vi "Setting.vi"() -> ()   [LabVIEW 2015]
uses:
  Control/Setting_Control_Main Action.ctl
  <vilib>/vision/Measure.llb/Edge Polarity.ctl
  <vilib>/Utility/miscctls.llb/LVPointTypeDef.ctl
  <vilib>/userdefined/High Color/IMAQdx.ctl
panel:
  out "狀態：":string
  out "群組：":string
  out "帳號：":string
  in  "物料名稱":enum16{"Tressel", "Diablo"}(ring)
  in  "匯入圖片":bool
  in  "邊參數L":T1={"Search Direction"=0, "Edge Polarity"=0, "Kernel Size"=3, "Width"=3, "Minimum Edge Strength"=10.0} {"Minimum Edge Strength" format="%.2f"; "Width" step=2; "Kernel Size" step=2; "Edge Polarity" items=["All Edges", "Rising Edges", "Falling Edges"]; "Search Direction" items=["Left to Right", "Right to Left", "Top to Bottom", "Bottom to Top"]}
  in  "邊參數R":T1={"Search Direction"=0, "Edge Polarity"=0, "Kernel Size"=3, "Width"=3, "Minimum Edge Strength"=10.0} {"Minimum Edge Strength" format="%.2f"; "Width" step=2; "Kernel Size" step=2; "Edge Polarity" items=["All Edges", "Rising Edges", "Falling Edges"]; "Search Direction" items=["Left to Right", "Right to Left", "Top to Bottom", "Bottom to Top"]}
  in  "樣本比對參數R":T3={"方法"=1, "分數"=800.0, "起始角度"=-5.0, "結束角度"=5.0} {"結束角度" min=-180 max=180 step=5; "方法" items=["快速比對"=1, "精準比對"=2]; "起始角度" min=-180 max=180 step=5}
  in  "樣本比對參數L":T3={"方法"=1, "分數"=800.0, "起始角度"=-5.0, "結束角度"=5.0} {"結束角度" min=-180 max=180 step=5; "方法" items=["快速比對"=1, "精準比對"=2]; "起始角度" min=-180 max=180 step=5}
  in  "確認檢測項目":bool
  in  "檢測項目":T4
  out "Patttern_R":T5(plugin-control)
  out "Patttern_L":T5(plugin-control)
  out "Image":T5(plugin-control)
  in  "離開":bool
  in  "連續測試":bool
  in  "單步測試":bool
  in  "連續取像":bool
  in  "取像":bool
  out "Set action":T6
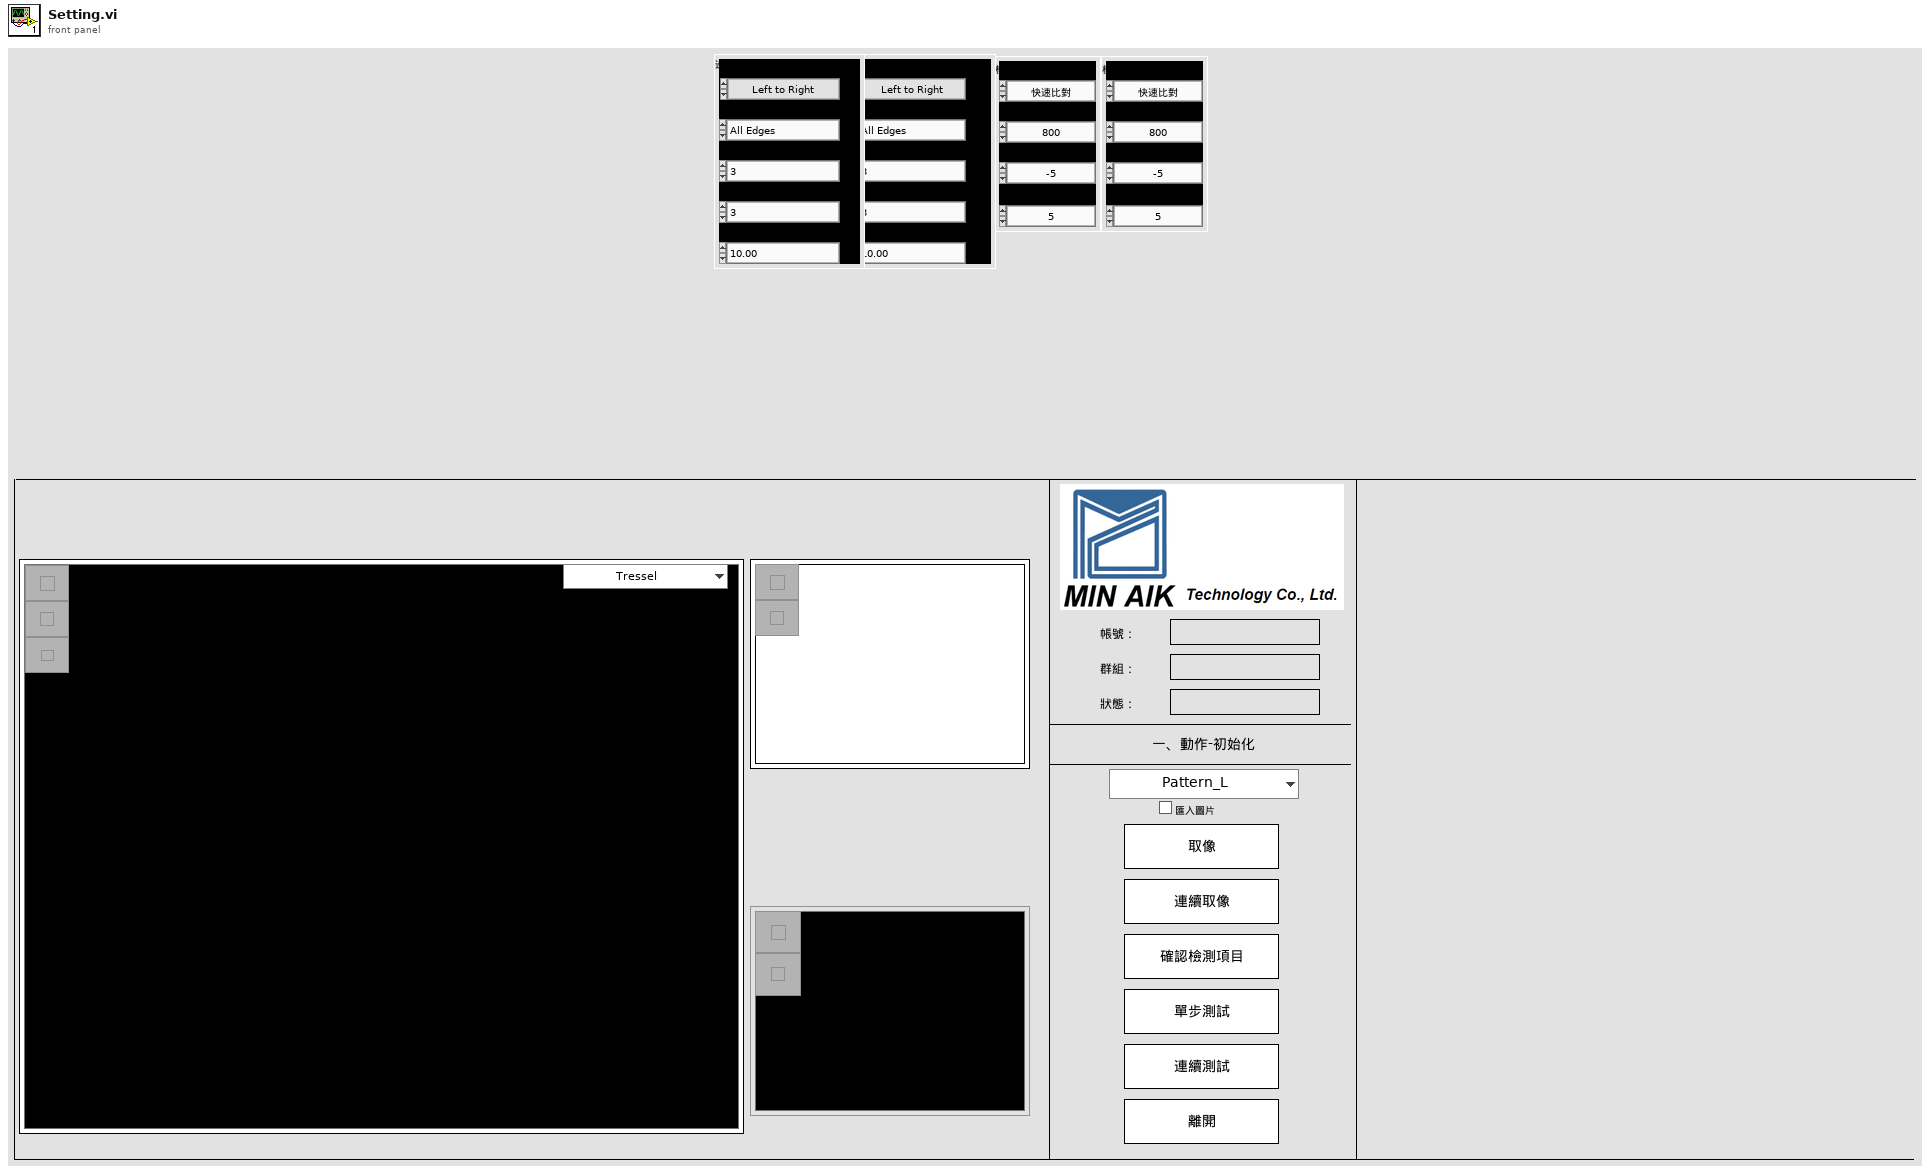
[diagram p1: front panel]
types:
  T1 = typedef "Setting_Control_Line Paremeter.ctl" = cluster{"Search Direction":u32, "Edge Polarity":T2, "Kernel Size":u32, "Width":u32, "Minimum Edge Strength":sgl}
  T2 = typedef "Edge Polarity.ctl" = u32
  T3 = typedef "Setting_Control_Pattern Paremeter.ctl" = cluster{"方法":u16, "分數":sgl, "起始角度":sgl, "結束角度":sgl}
  T4 = typedef "Setting_Control_檢測項目.ctl" = enum16{"Pattern_L", "Match_L", "Pattern_R", "Match_R", "找邊_L", "找邊R"}
  T5 = typedef "IMAQ Image.ctl" = refnum<image>
  T6 = typedef "Setting_Control_Main Action.ctl" = enum16{"一、動作-初始化", "二、動作-單次取像", "三、動作-連續取像", "四、動作-單步測試", "五、動作-連續測試", "六、動作-離開", "1.0 功能-IO控制", "       1.1 IO-初始化", "       1.2 Set Point(EOT On)", "       1.3Set Point(EOT Off)", "       1.4Get Point(SOT)", "2.0功能-相機控制", "       2.1相機-初始化", "       2.2相機-取像", "       2.3相機-關閉", "3.0功能-影像控制", "       3.1影像-初始化", "       3.2影像-更新影像", "       3.3影像-儲存影像", "4.0功能-檢測", "       4.1檢測-初始化", "      4.2浪代-浪代", "             4.2.1浪代-Pattern_L", "             4.2.2浪代-Match_L", "             4.2.3浪代-Pattern_R", "             4.2.4浪代-Match_R", "             4.2.5檢測-找邊_L", "             4.2.6檢測-找邊_R", "5.0功能-雷射控制", "      5.1雷射-初始化", "      5.2雷射-寫入數值", "      5.3雷射-讀出數值", "      5.4雷射-雷射觸發", "      5.5雷射-關閉", "6.0功能-檔案", "       6.1檔案-初始化", "       6.2檔案-儲存檔案", "       6.3檔案-開啟檔案", "7.0 錯誤", "8.0等待", "       8.1等待(計算時間)", "9.0離開", "10.0功能-機台驗證", "      10.1機台驗證-初始化", "      10.2機台驗證-檢測", "11.0對話視窗"}
  T7 = typedef "LVPointTypeDef.ctl" = cluster{"Horizontal":i16, "Vertical":i16}
  T8 = typedef "IMAQdx.ctl" = refnum<k21>
  T9 = typedef "action_camera.ctl" = enum16{"初始化", "取像", "匯入影像", "結束"}
  T10 = typedef "Image action.ctl" = enum16{"初始化", "創造記憶體", "寫入圖片", "讀取圖片", "刪除圖片", "等待"}
  T11 = cluster{"邊參數R":T1, "ROI":cluster{"Global Rectangle":i32[], "Contours":cluster{"Contour Type":u32, "ROI Type":u32, "Points":i32[]}[]}}
  T12 = cluster{"邊參數L":T1, "ROI":cluster{"Global Rectangle":i32[], "Contours":cluster{"Contour Type":u32, "ROI Type":u32, "Points":i32[]}[]}}
  T13 = typedef "IMAQ Coordinate System" = cluster{"Reference System":cluster{"Origin":cluster{"X":sgl, "Y":sgl}, "Angle (deg)":sgl, "Axis Reference":u32}, "Measurement System":cluster{"Origin":cluster{"X":sgl, "Y":sgl}, "Angle (deg)":sgl, "Axis Reference":u32}}
  T14 = cluster{"ROI":cluster{"Global Rectangle":i32[], "Contours":cluster{"Contour Type":u32, "ROI Type":u32, "Points":i32[]}[]}, "樣本比對參數R":T3, "Coordinate System Out":T13}
  T15 = cluster{"樣本比對參數L":T3, "ROI":cluster{"Global Rectangle":i32[], "Contours":cluster{"Contour Type":u32, "ROI Type":u32, "Points":i32[]}[]}, "Coordinate System Out":T13}
  T16 = typedef "Action_Data.ctl" = enum16{"Initialize", "Get Data", "Set Data", "Delete Data", "Idle"}
  T17 = typedef "Image Type" = u32
  T18 = cluster{"Global Rectangle":i32[], "Contours":cluster{"Contour Type":u32, "ROI Type":u32, "Points":i32[]}[]}
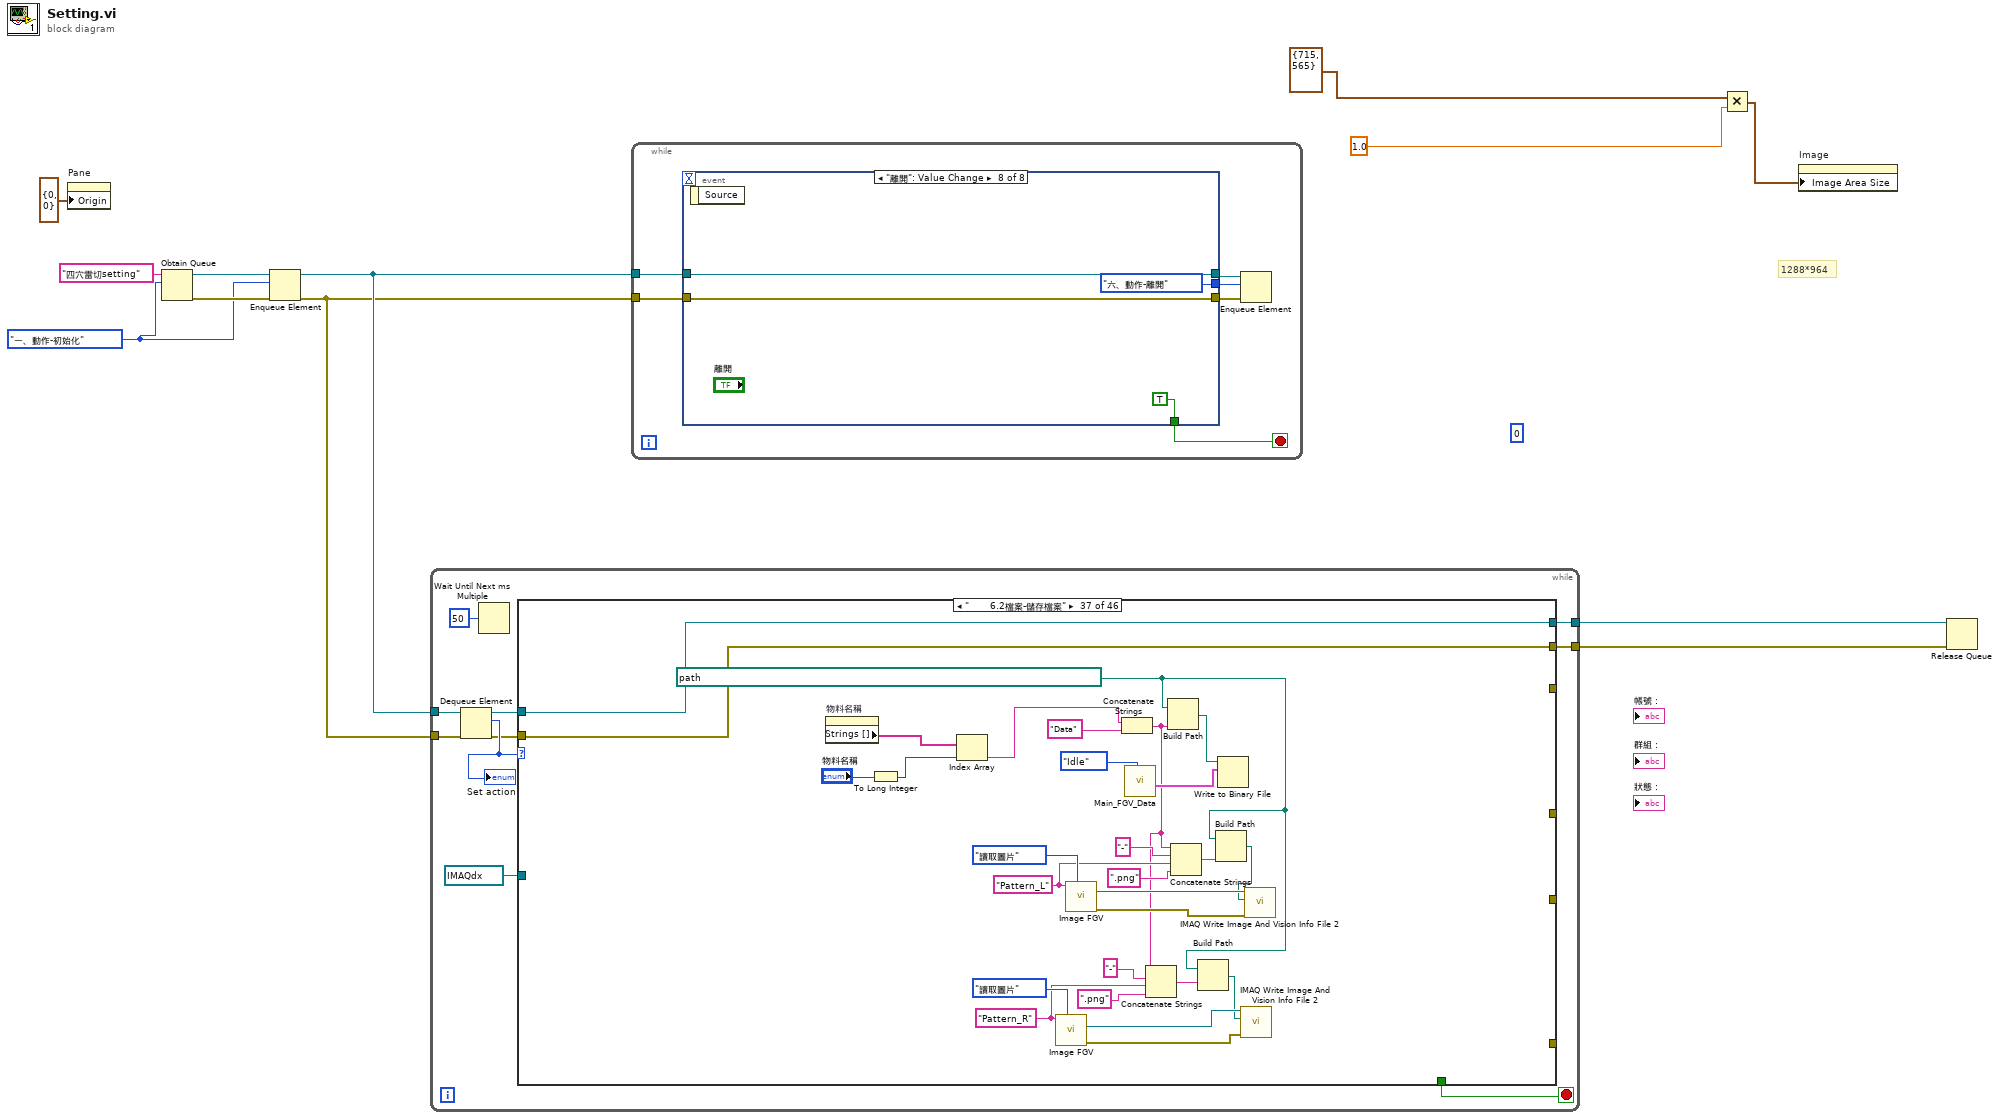
[diagram p0: block diagram]
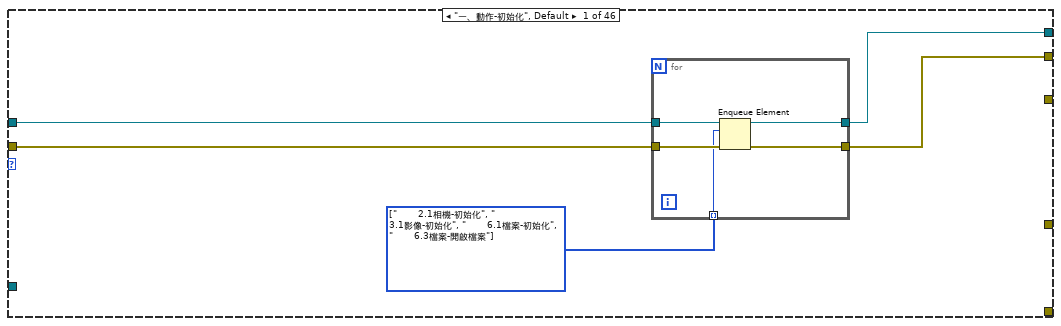
[diagram p2: hidden frame]
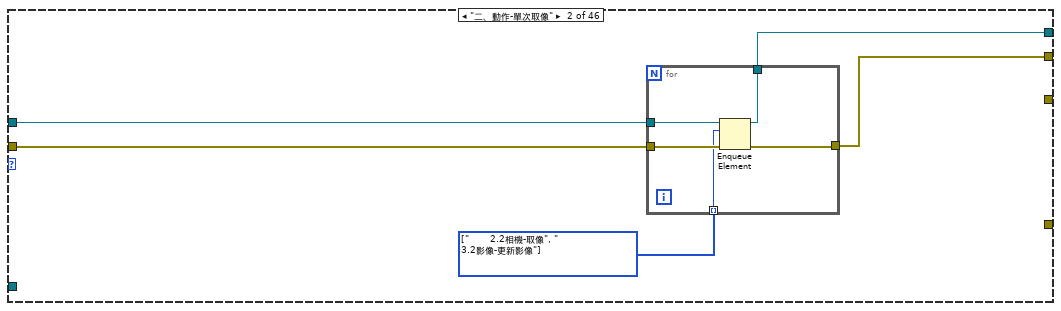
[diagram p3: hidden frame]
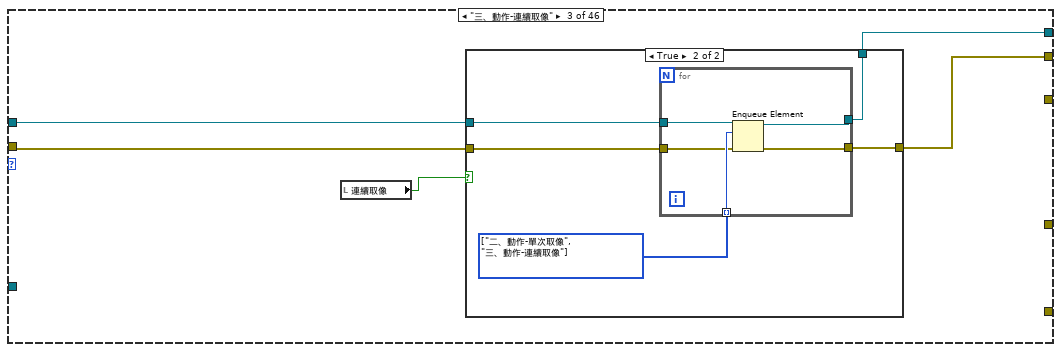
[diagram p4: hidden frame]
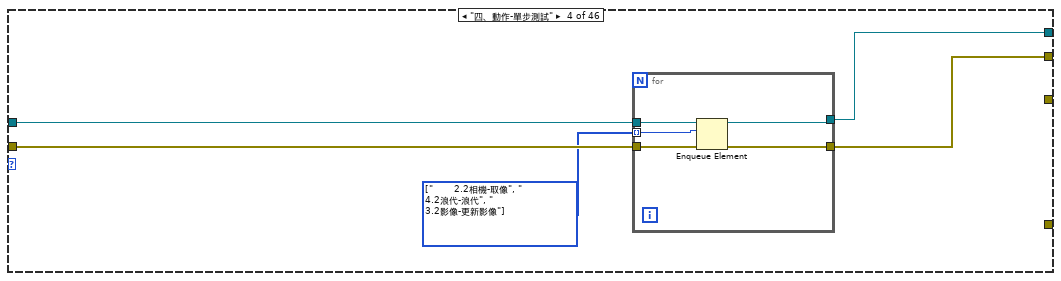
[diagram p6: hidden frame]
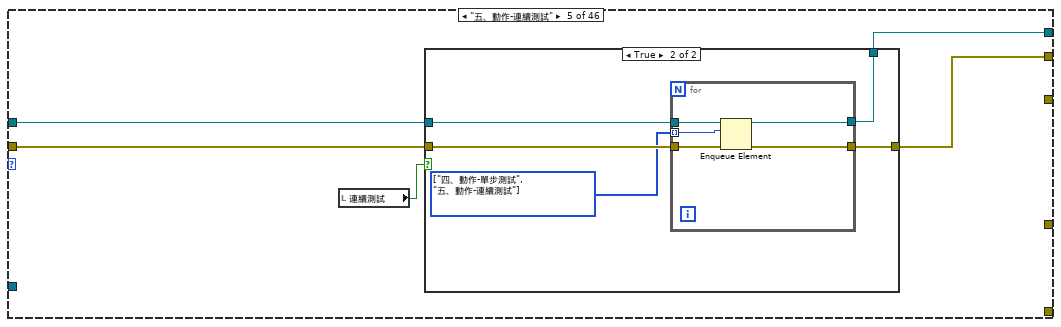
[diagram p7: hidden frame]
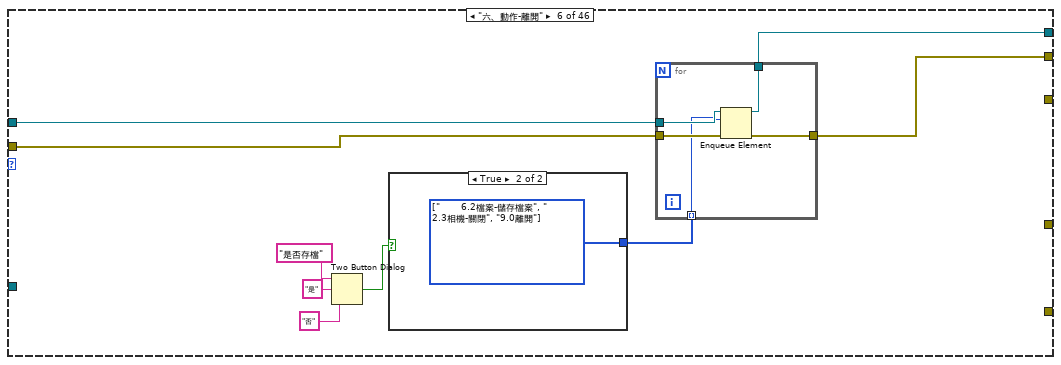
[diagram p9: hidden frame]
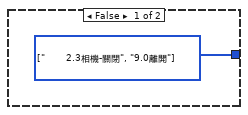
[diagram p10: hidden frame]
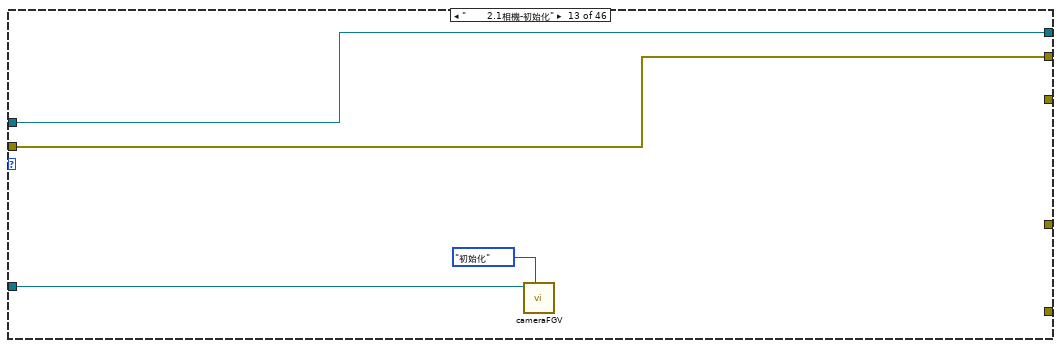
[diagram p17: hidden frame]
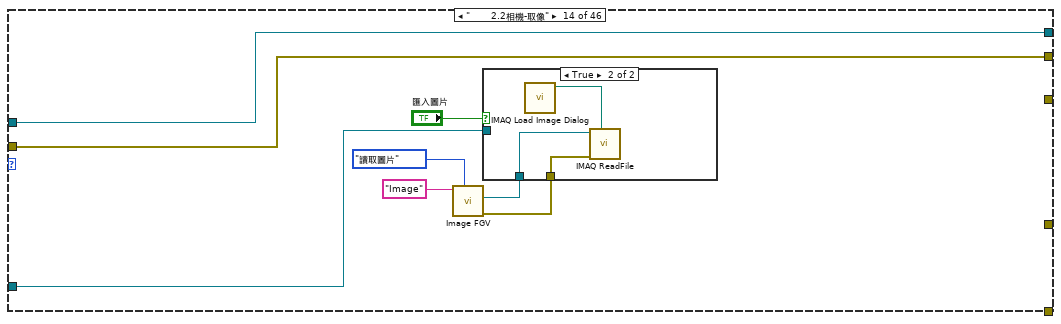
[diagram p18: hidden frame]
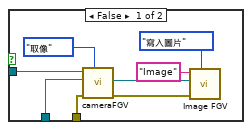
[diagram p19: hidden frame]
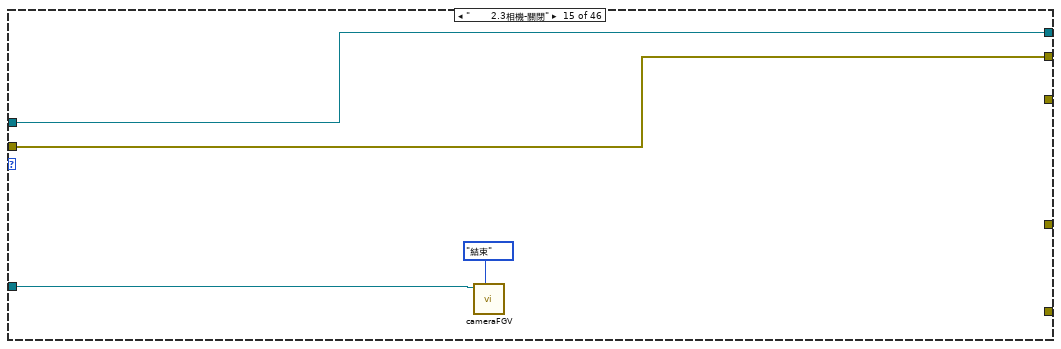
[diagram p20: hidden frame]
diagram:
  (unwired) 0
  w9 = Setting_Control_Main_Action."一、動作-初始化" ("element")
  # "1288*964"
  n1 = property on="Pane" class="Pane"("Origin"=T7 {"Horizontal"=0, "Vertical"=0}) -> ()  [unwired: 2 in, 2 out]
  n2 = Obtain Queue(name (unnamed)="四穴雷切setting", element data type=w9) -> (queue out=w11:refnum<queue>, error out=w10:errorcluster)  [unwired: 3 in, 1 out]
  n3 = Enqueue Element(queue=w11, element=w9, error in (no error)=w10) -> (queue out=w8:refnum<queue>, error out=w7:errorcluster)  [unwired: 1 in, 1 out]
  n4 = while {
    tunnel: w8 -> [w22]
    tunnel: w7 -> [w21]
    tunnel: [w16] -> w6
    tunnel: [w15] -> w5
    stop <- w20 stop-if-true
    n5 = Dequeue Element(queue=w22, error in (no error)=w21) -> (queue out=w18:refnum<queue>, element=w19:T6, error out=w17:errorcluster)  [unwired: 1 in, 1 out]
    "Set action" <- w19
    n6 = Wait Until Next ms Multiple(millisecond multiple=u32 50) -> ()  [unwired: 1 out]
    n7 = case shown="\"       6.2檔案-儲存檔案\"" w19 {
      tunnel: [_ _ _ _ _ _ _ _ _ _ _ _ _ _ _ _ _ _ _ _ _ _ _ _ _ _ _ _ _ _ _ _ _ _ _ _ _ _ _ _ _ TRUE _ _ _ _] -> w20
      tunnel: w18 -> [w24 w37 w47 w64 w74 w95 w104 w106 w108 w110 w112 w114 w117 w121 w141 w143 w147 w167 w169 w171 w173 w203 w237 w253 w265 w290 w317 w323 w338 w340 w342 w344 w346 w348 w350 w353 w381 w404 w418 w420 w422 w424 w427 w429 w431 w433]
      tunnel: w17 -> [w27 w36 w46 w63 w73 w94 w103 w105 w107 w109 w111 w113 w115 w120 w140 w142 w144 w156 w168 w170 w172 w202 w235 w251 w264 w289 w316 w320 w337 w339 w341 w343 w345 w347 w349 w352 w380 w403 w417 w419 w421 w423 w426 w428 w430 w432]
      tunnel: [w25 w34 w45 w62 w72 w93 w104 w106 w108 w110 w112 w114 w117 w121 w141 w143 w147 w167 w169 w171 w173 w203 w236 w252 w266 w288 w315 w322 w338 w340 w342 w344 w346 w348 w350 w353 w381 w402 w418 w420 w422 w424 w427 w429 w431 w433] -> w16
      tunnel: [w26 w35 w44 w61 w71 w92 w103 w105 w107 w109 w111 w113 w115 w120 w140 w142 w144 w156 w168 w170 w172 w202 w234 w250 w263 w287 w314 w319 w337 w339 w341 w343 w345 w347 w349 w352 w380 w401 w417 w419 w421 w423 w426 w428 w430 w432] -> w15
      tunnel: T8 "cam0" ("Session In") -> [_ _ _ _ _ _ _ _ _ _ _ _ w116 w122 w139 _ _ _ _ _ _ _ _ _ _ _ _ _ _ _ _ _ _ _ _ _ _ _ _ _ _ _ _ _ _ _]
      tunnel: [_ _ _ _ _ _ _ _ _ _ _ _ _ _ _ _ _ _ _ _ _ _ _ _ _ _ _ _ _ _ _ _ _ _ _ _ _ w397 _ _ _ _ _ _ _ _] -> _
      tunnel: [_ _ _ _ _ _ _ _ _ _ _ _ _ _ _ _ _ _ _ _ _ _ _ _ _ _ _ _ _ _ _ _ _ _ _ _ _ w396 _ _ _ _ _ _ _ _] -> _
      tunnel: [_ _ _ _ _ _ _ _ _ _ _ _ _ _ _ _ _ _ _ _ _ _ _ _ _ _ _ _ _ _ _ _ _ _ _ _ _ w383 _ _ _ _ _ _ _ _] -> _
      tunnel: [_ _ _ _ _ _ _ _ _ _ _ _ _ _ _ _ _ _ _ _ _ _ _ _ _ _ _ _ _ _ _ _ _ _ _ _ _ w382 _ _ _ _ _ _ _ _] -> _
      frame "一、動作-初始化", Default {
        w23 = T6[] [enum."       2.1相機-初始化", enum."       3.1影像-初始化", enum."       6.1檔案-初始化", enum."       6.3檔案-開啟檔案"] items=["一、動作-初始化", "二、動作-單次取像", "三、動作-連續取像", "四、動作-單步測試", "五、動作-連續測試", "六、動作-離開", "1.0 功能-IO控制", "       1.1 IO-初始化", "       1.2 Set Point(EOT On)", "       1.3Set Point(EOT Off)", "       1.4Get Point(SOT)", "2.0功能-相機控制", "       2.1相機-初始化", "       2.2相機-取像", "       2.3相機-關閉", "3.0功能-影像控制", "       3.1影像-初始化", "       3.2影像-更新影像", "       3.3影像-儲存影像", "4.0功能-檢測", "       4.1檢測-初始化", "      4.2浪代-浪代", "             4.2.1浪代-Pattern_L", "             4.2.2浪代-Match_L", "             4.2.3浪代-Pattern_R", "             4.2.4浪代-Match_R", "             4.2.5檢測-找邊_L", "             4.2.6檢測-找邊_R", "5.0功能-雷射控制", "      5.1雷射-初始化", "      5.2雷射-寫入數值", "      5.3雷射-讀出數值", "      5.4雷射-雷射觸發", "      5.5雷射-關閉", "6.0功能-檔案", "       6.1檔案-初始化", "       6.2檔案-儲存檔案", "       6.3檔案-開啟檔案", "7.0 錯誤", "8.0等待", "       8.1等待(計算時間)", "9.0離開", "10.0功能-機台驗證", "      10.1機台驗證-初始化", "      10.2機台驗證-檢測", "11.0對話視窗"]
        n8 = for {
          tunnel: w24 -> [w32]
          tunnel: w27 -> [w31]
          tunnel: [w30] -> w26
          tunnel: [w29] -> w25
          tunnel: w23 -> [w28] mode=indexing
          n9 = Enqueue Element(queue=w32, element=w28, error in (no error)=w31) -> (queue out=w29:refnum<queue>, error out=w30:errorcluster)  [unwired: 1 in, 1 out]
        }
      }
      frame "二、動作-單次取像" {
        w33 = T6[] [enum."       2.2相機-取像", enum."       3.2影像-更新影像"] items=["一、動作-初始化", "二、動作-單次取像", "三、動作-連續取像", "四、動作-單步測試", "五、動作-連續測試", "六、動作-離開", "1.0 功能-IO控制", "       1.1 IO-初始化", "       1.2 Set Point(EOT On)", "       1.3Set Point(EOT Off)", "       1.4Get Point(SOT)", "2.0功能-相機控制", "       2.1相機-初始化", "       2.2相機-取像", "       2.3相機-關閉", "3.0功能-影像控制", "       3.1影像-初始化", "       3.2影像-更新影像", "       3.3影像-儲存影像", "4.0功能-檢測", "       4.1檢測-初始化", "      4.2浪代-浪代", "             4.2.1浪代-Pattern_L", "             4.2.2浪代-Match_L", "             4.2.3浪代-Pattern_R", "             4.2.4浪代-Match_R", "             4.2.5檢測-找邊_L", "             4.2.6檢測-找邊_R", "5.0功能-雷射控制", "      5.1雷射-初始化", "      5.2雷射-寫入數值", "      5.3雷射-讀出數值", "      5.4雷射-雷射觸發", "      5.5雷射-關閉", "6.0功能-檔案", "       6.1檔案-初始化", "       6.2檔案-儲存檔案", "       6.3檔案-開啟檔案", "7.0 錯誤", "8.0等待", "       8.1等待(計算時間)", "9.0離開", "10.0功能-機台驗證", "      10.1機台驗證-初始化", "      10.2機台驗證-檢測", "11.0對話視窗"]
        n10 = for {
          tunnel: w37 -> [w42]
          tunnel: w36 -> [w41]
          tunnel: [w40] -> w35
          tunnel: [w39] -> w34
          tunnel: w33 -> [w38] mode=indexing
          n11 = Enqueue Element(queue=w42, element=w38, error in (no error)=w41) -> (queue out=w39:refnum<queue>, error out=w40:errorcluster)  [unwired: 1 in, 1 out]
        }
      }
      frame "三、動作-連續取像" {
        n12 = local read "連續取像"() -> (w43:bool)
        n13 = case shown="True" w43 {
          tunnel: w47 -> [w49 w53]
          tunnel: w46 -> [w48 w52]
          tunnel: [w49 w51] -> w45
          tunnel: [w48 w50] -> w44
          frame False {
          }
          frame True {
            w54 = T6[] [enum."二、動作-單次取像", enum."三、動作-連續取像"] items=["一、動作-初始化", "二、動作-單次取像", "三、動作-連續取像", "四、動作-單步測試", "五、動作-連續測試", "六、動作-離開", "1.0 功能-IO控制", "       1.1 IO-初始化", "       1.2 Set Point(EOT On)", "       1.3Set Point(EOT Off)", "       1.4Get Point(SOT)", "2.0功能-相機控制", "       2.1相機-初始化", "       2.2相機-取像", "       2.3相機-關閉", "3.0功能-影像控制", "       3.1影像-初始化", "       3.2影像-更新影像", "       3.3影像-儲存影像", "4.0功能-檢測", "       4.1檢測-初始化", "      4.2浪代-浪代", "             4.2.1浪代-Pattern_L", "             4.2.2浪代-Match_L", "             4.2.3浪代-Pattern_R", "             4.2.4浪代-Match_R", "             4.2.5檢測-找邊_L", "             4.2.6檢測-找邊_R", "5.0功能-雷射控制", "      5.1雷射-初始化", "      5.2雷射-寫入數值", "      5.3雷射-讀出數值", "      5.4雷射-雷射觸發", "      5.5雷射-關閉", "6.0功能-檔案", "       6.1檔案-初始化", "       6.2檔案-儲存檔案", "       6.3檔案-開啟檔案", "7.0 錯誤", "8.0等待", "       8.1等待(計算時間)", "9.0離開", "10.0功能-機台驗證", "      10.1機台驗證-初始化", "      10.2機台驗證-檢測", "11.0對話視窗"]
            n14 = for {
              tunnel: [w59] -> w50
              tunnel: [w58] -> w51
              tunnel: w54 -> [w57] mode=indexing
              tunnel: w53 -> [w56]
              tunnel: w52 -> [w55]
              n15 = Enqueue Element(queue=w56, element=w57, error in (no error)=w55) -> (queue out=w58:refnum<queue>, error out=w59:errorcluster)  [unwired: 1 in, 1 out]
            }
          }
        }
      }
      frame "四、動作-單步測試" {
        w60 = T6[] [enum."       2.2相機-取像", enum."      4.2浪代-浪代", enum."       3.2影像-更新影像"] items=["一、動作-初始化", "二、動作-單次取像", "三、動作-連續取像", "四、動作-單步測試", "五、動作-連續測試", "六、動作-離開", "1.0 功能-IO控制", "       1.1 IO-初始化", "       1.2 Set Point(EOT On)", "       1.3Set Point(EOT Off)", "       1.4Get Point(SOT)", "2.0功能-相機控制", "       2.1相機-初始化", "       2.2相機-取像", "       2.3相機-關閉", "3.0功能-影像控制", "       3.1影像-初始化", "       3.2影像-更新影像", "       3.3影像-儲存影像", "4.0功能-檢測", "       4.1檢測-初始化", "      4.2浪代-浪代", "             4.2.1浪代-Pattern_L", "             4.2.2浪代-Match_L", "             4.2.3浪代-Pattern_R", "             4.2.4浪代-Match_R", "             4.2.5檢測-找邊_L", "             4.2.6檢測-找邊_R", "5.0功能-雷射控制", "      5.1雷射-初始化", "      5.2雷射-寫入數值", "      5.3雷射-讀出數值", "      5.4雷射-雷射觸發", "      5.5雷射-關閉", "6.0功能-檔案", "       6.1檔案-初始化", "       6.2檔案-儲存檔案", "       6.3檔案-開啟檔案", "7.0 錯誤", "8.0等待", "       8.1等待(計算時間)", "9.0離開", "10.0功能-機台驗證", "      10.1機台驗證-初始化", "      10.2機台驗證-檢測", "11.0對話視窗"]
        n16 = for {
          tunnel: w64 -> [w69]
          tunnel: w63 -> [w68]
          tunnel: [w67] -> w62
          tunnel: [w66] -> w61
          tunnel: w60 -> [w65] mode=indexing
          n17 = Enqueue Element(queue=w69, element=w65, error in (no error)=w68) -> (queue out=w67:refnum<queue>, error out=w66:errorcluster)  [unwired: 1 in, 1 out]
        }
      }
      frame "五、動作-連續測試" {
        n18 = local read "連續測試"() -> (w70:bool)
        n19 = case shown="True" w70 {
          tunnel: w74 -> [w76 w81]
          tunnel: w73 -> [w75 w80]
          tunnel: [w76 w79] -> w72
          tunnel: [w75 w78] -> w71
          frame False {
          }
          frame True {
            w77 = T6[] [enum."四、動作-單步測試", enum."五、動作-連續測試"] items=["一、動作-初始化", "二、動作-單次取像", "三、動作-連續取像", "四、動作-單步測試", "五、動作-連續測試", "六、動作-離開", "1.0 功能-IO控制", "       1.1 IO-初始化", "       1.2 Set Point(EOT On)", "       1.3Set Point(EOT Off)", "       1.4Get Point(SOT)", "2.0功能-相機控制", "       2.1相機-初始化", "       2.2相機-取像", "       2.3相機-關閉", "3.0功能-影像控制", "       3.1影像-初始化", "       3.2影像-更新影像", "       3.3影像-儲存影像", "4.0功能-檢測", "       4.1檢測-初始化", "      4.2浪代-浪代", "             4.2.1浪代-Pattern_L", "             4.2.2浪代-Match_L", "             4.2.3浪代-Pattern_R", "             4.2.4浪代-Match_R", "             4.2.5檢測-找邊_L", "             4.2.6檢測-找邊_R", "5.0功能-雷射控制", "      5.1雷射-初始化", "      5.2雷射-寫入數值", "      5.3雷射-讀出數值", "      5.4雷射-雷射觸發", "      5.5雷射-關閉", "6.0功能-檔案", "       6.1檔案-初始化", "       6.2檔案-儲存檔案", "       6.3檔案-開啟檔案", "7.0 錯誤", "8.0等待", "       8.1等待(計算時間)", "9.0離開", "10.0功能-機台驗證", "      10.1機台驗證-初始化", "      10.2機台驗證-檢測", "11.0對話視窗"]
            n20 = for {
              tunnel: w81 -> [w86]
              tunnel: w80 -> [w85]
              tunnel: [w84] -> w79
              tunnel: [w83] -> w78
              tunnel: w77 -> [w82] mode=indexing
              n21 = Enqueue Element(queue=w86, element=w82, error in (no error)=w85) -> (queue out=w84:refnum<queue>, error out=w83:errorcluster)  [unwired: 1 in, 1 out]
            }
          }
        }
      }
      frame "六、動作-離開" {
        n22 = Two Button Dialog(message="是否存檔", 1:"否" ("F button name (\"Cancel\")"), 2:"是" ("T button name (\"OK\")")) -> (T button?=w91:bool)
        n23 = case shown="True" w91 {
          tunnel: [w96 w97] -> w87
          frame False {
            w96 = T6[] [enum."       2.3相機-關閉", enum."9.0離開"] items=["一、動作-初始化", "二、動作-單次取像", "三、動作-連續取像", "四、動作-單步測試", "五、動作-連續測試", "六、動作-離開", "1.0 功能-IO控制", "       1.1 IO-初始化", "       1.2 Set Point(EOT On)", "       1.3Set Point(EOT Off)", "       1.4Get Point(SOT)", "2.0功能-相機控制", "       2.1相機-初始化", "       2.2相機-取像", "       2.3相機-關閉", "3.0功能-影像控制", "       3.1影像-初始化", "       3.2影像-更新影像", "       3.3影像-儲存影像", "4.0功能-檢測", "       4.1檢測-初始化", "      4.2浪代-浪代", "             4.2.1浪代-Pattern_L", "             4.2.2浪代-Match_L", "             4.2.3浪代-Pattern_R", "             4.2.4浪代-Match_R", "             4.2.5檢測-找邊_L", "             4.2.6檢測-找邊_R", "5.0功能-雷射控制", "      5.1雷射-初始化", "      5.2雷射-寫入數值", "      5.3雷射-讀出數值", "      5.4雷射-雷射觸發", "      5.5雷射-關閉", "6.0功能-檔案", "       6.1檔案-初始化", "       6.2檔案-儲存檔案", "       6.3檔案-開啟檔案", "7.0 錯誤", "8.0等待", "       8.1等待(計算時間)", "9.0離開", "10.0功能-機台驗證", "      10.1機台驗證-初始化", "      10.2機台驗證-檢測", "11.0對話視窗"]
          }
          frame True {
            w97 = T6[] [enum."       6.2檔案-儲存檔案", enum."       2.3相機-關閉", enum."9.0離開"] items=["一、動作-初始化", "二、動作-單次取像", "三、動作-連續取像", "四、動作-單步測試", "五、動作-連續測試", "六、動作-離開", "1.0 功能-IO控制", "       1.1 IO-初始化", "       1.2 Set Point(EOT On)", "       1.3Set Point(EOT Off)", "       1.4Get Point(SOT)", "2.0功能-相機控制", "       2.1相機-初始化", "       2.2相機-取像", "       2.3相機-關閉", "3.0功能-影像控制", "       3.1影像-初始化", "       3.2影像-更新影像", "       3.3影像-儲存影像", "4.0功能-檢測", "       4.1檢測-初始化", "      4.2浪代-浪代", "             4.2.1浪代-Pattern_L", "             4.2.2浪代-Match_L", "             4.2.3浪代-Pattern_R", "             4.2.4浪代-Match_R", "             4.2.5檢測-找邊_L", "             4.2.6檢測-找邊_R", "5.0功能-雷射控制", "      5.1雷射-初始化", "      5.2雷射-寫入數值", "      5.3雷射-讀出數值", "      5.4雷射-雷射觸發", "      5.5雷射-關閉", "6.0功能-檔案", "       6.1檔案-初始化", "       6.2檔案-儲存檔案", "       6.3檔案-開啟檔案", "7.0 錯誤", "8.0等待", "       8.1等待(計算時間)", "9.0離開", "10.0功能-機台驗證", "      10.1機台驗證-初始化", "      10.2機台驗證-檢測", "11.0對話視窗"]
          }
        }
        n24 = for {
          tunnel: w95 -> [w102]
          tunnel: w94 -> [w101]
          tunnel: [w100] -> w93
          tunnel: [w99] -> w92
          tunnel: w87 -> [w98] mode=indexing
          n25 = Enqueue Element(queue=w102, element=w98, error in (no error)=w101) -> (queue out=w100:refnum<queue>, error out=w99:errorcluster)  [unwired: 1 in, 1 out]
        }
      }
      frame "1.0 功能-IO控制" {
      }
      frame "       1.1 IO-初始化" {
      }
      frame "       1.2 Set Point(EOT On)" {
      }
      frame "       1.3Set Point(EOT Off)" {
      }
      frame "       1.4Get Point(SOT)" {
      }
      frame "2.0功能-相機控制" {
      }
      frame "       2.1相機-初始化" {
        n26 = call "cameraFGV.vi"("action_camera"=action_camera."初始化", "Session In"=w116) -> ()  [unwired: 7 in, 3 out]
      }
      frame "       2.2相機-取像" {
        n27 = call "Image FGV.vi"("Image action"=Image_action."讀取圖片", "圖片名稱"="Image") -> ("error out"=w123:errorcluster, "Image Out"=w124:T5)  [unwired: 8 in]
        n28 = case shown="True" "匯入圖片" {
          tunnel: w124 -> [w134 w137]
          tunnel: w123 -> [w133 w136]
          tunnel: w122 -> [w132 _]
          frame False {
            n29 = call "cameraFGV.vi"("action_camera"=action_camera."取像", "error constant"=w133, "Image In"=w134, "Session In"=w132) -> ("error constant 2"=w131:errorcluster, "Image Out"=w130:T5)  [unwired: 5 in, 1 out]
            n30 = call "Image FGV.vi"("Image action"=Image_action."寫入圖片", "error in (no error)"=w131, "Image In"=w130, "圖片名稱"="Image") -> ()  [unwired: 6 in, 2 out]
          }
          frame True {
            n31 = call "IMAQ Load Image Dialog"() -> ("Path"=w135:path)  [unwired: 9 in, 2 out]
            n32 = call "IMAQ ReadFile"("File Path"=w135, "error in (no error)"=w136, "Image"=w137) -> ()  [unwired: 4 in, 5 out]
          }
        }
      }
      frame "       2.3相機-關閉" {
        n33 = call "cameraFGV.vi"("action_camera"=action_camera."結束", "Session In"=w139) -> ()  [unwired: 7 in, 3 out]
      }
      frame "3.0功能-影像控制" {
      }
      frame "       3.1影像-初始化" {
        w145 = T17[] [0, 0, 0] items=["Grayscale (U8)", "Grayscale (I16)", "Grayscale (SGL)", "Complex (CSG)", "RGB (U32)", "HSL (U32)", "RGB (U64)", "Grayscale (U16)"]
        n34 = call "Image FGV.vi"("Image action"=Image_action."初始化") -> ("error out"=w148:errorcluster)  [unwired: 9 in, 1 out]
        n35 = for {
          tunnel: w148 -> [w153]
          tunnel: string[] ["Image", "Pattern_L", "Pattern_R"] -> [w151] mode=indexing
          tunnel: w145 -> [w150] mode=indexing
          n36 = call "Image FGV.vi"("Image action"=Image_action."創造記憶體", "error in (no error)"=w153, "Image Type"=w150, "圖片名稱"=w151) -> ()  [unwired: 6 in, 2 out]
        }
      }
      frame "       3.2影像-更新影像" {
        n37 = call "Image FGV.vi"("Image action"=Image_action."讀取圖片", "圖片名稱"="Pattern_L") -> ("Image Out"=→"Patttern_L":T5)  [unwired: 8 in, 1 out]
        n38 = call "Image FGV.vi"("Image action"=Image_action."讀取圖片", "圖片名稱"="Pattern_R") -> ("Image Out"=→"Patttern_R":T5)  [unwired: 8 in, 1 out]
        n39 = call "Image FGV.vi"("Image action"=Image_action."讀取圖片", "圖片名稱"="Image") -> ("Image Out"=→"Image":T5)  [unwired: 8 in, 1 out]
        n40 = property on="Patttern_L" class="ImageControl"("Zoom to Fit Mode"=TRUE) -> ()  [unwired: 2 in, 2 out]
        n41 = property on="Image" class="ImageControl"("Zoom to Fit Mode"=TRUE) -> ()  [unwired: 2 in, 2 out]
        n42 = property on="Patttern_R" class="ImageControl"("Zoom to Fit Mode"=TRUE) -> ()  [unwired: 2 in, 2 out]
      }
      frame "       3.3影像-儲存影像" {
      }
      frame "4.0功能-檢測" {
      }
      frame "       4.1檢測-初始化" {
      }
      frame "      4.2浪代-浪代" {
        w210 = u16 1 items=["Find Reference", "Update CoordSys"] ("Mode")
        w220 = u16 1 items=["Find Reference", "Update CoordSys"] ("Mode")
        n43 = call "Main_FGV_Data.vi"("Action_Data"=Action_Data."Idle") -> ("Data Array out"=w191:cluster{"Data name":string, "Data":variant}[])  [unwired: 9 in, 1 out]
        n44 = Index Array(array=w191, index #1=0 ("index"), index #2=1 ("index"), index #3=2 ("index"), index #4=3 ("index")) -> (element #1=w215:cluster{"Data name":string, "Data":variant}, element #2=w208:cluster{"Data name":string, "Data":variant}, element #3=w197:cluster{"Data name":string, "Data":variant}, element #4=w182:cluster{"Data name":string, "Data":variant})
        n45 = Unbundle By Name(w215) -> ("Data"=w214:variant)
        n46 = Unbundle By Name(w208) -> ("Data"=w207:variant)
        n47 = Unbundle By Name(w197) -> ("Data"=w196:variant)
        n48 = Unbundle By Name(w182) -> ("Data"=w180:variant)
        n49 = call "Image FGV.vi"("Image action"=Image_action."讀取圖片", "圖片名稱"="Pattern_L") -> ("Image Out"=w219:T5)  [unwired: 8 in, 1 out]
        n50 = call "Image FGV.vi"("Image action"=Image_action."讀取圖片", "圖片名稱"="Image") -> ("Image Out"=w201:T5)  [unwired: 8 in, 1 out]
        n51 = Variant To Data(type=T15 {"樣本比對參數L"={"方法"=0, "分數"=0.0, "起始角度"=0.0, "結束角度"=0.0}, "ROI"={"Global Rectangle"=[], "Contours"=[]}, "Coordinate System Out"={"Reference System"={"Origin"={"X"=0.0, "Y"=0.0}, "Angle (deg)"=0.0, "Axis Reference"=0}, "Measurement System"={"Origin"={"X"=0.0, "Y"=0.0}, "Angle (deg)"=0.0, "Axis Reference"=0}}} ("output cluster"), Variant=w214) -> (data=w218:T15)  [unwired: 1 in, 1 out]
        n52 = Variant To Data(type=T11 {"邊參數R"={"Search Direction"=0, "Edge Polarity"=0, "Kernel Size"=0, "Width"=0, "Minimum Edge Strength"=0.0}, "ROI"={"Global Rectangle"=[], "Contours"=[]}} ("output cluster"), Variant=w180) -> (data=w177:T11)  [unwired: 1 in, 1 out]
        n53 = Variant To Data(type=T12 {"邊參數L"={"Search Direction"=0, "Edge Polarity"=0, "Kernel Size"=0, "Width"=0, "Minimum Edge Strength"=0.0}, "ROI"={"Global Rectangle"=[], "Contours"=[]}} ("output cluster"), Variant=w196) -> (data=w195:T12)  [unwired: 1 in, 1 out]
        n54 = Unbundle(w218) -> ("樣本比對參數L"=w188:T3, "ROI"=w217:T18, "Coordinate System Out"=w190:T13)
        n55 = call "浪代_Match_Sub.vi"("樣本比對參數"=w188, "ROI Descriptor"=w217, "Mode"=w220, "Coordinate System In"=w190, "Template Image"=w219, "Image"=w201) -> ("error out"=w209:errorcluster, "Coordinate System Out"=w193:T13)  [unwired: 3 in, 1 out]
        n56 = Variant To Data(type=T14 {"ROI"={"Global Rectangle"=[], "Contours"=[]}, "樣本比對參數R"={"方法"=0, "分數"=0.0, "起始角度"=0.0, "結束角度"=0.0}, "Coordinate System Out"={"Reference System"={"Origin"={"X"=0.0, "Y"=0.0}, "Angle (deg)"=0.0, "Axis Reference"=0}, "Measurement System"={"Origin"={"X"=0.0, "Y"=0.0}, "Angle (deg)"=0.0, "Axis Reference"=0}}} ("output cluster"), Variant=w207) -> (data=w206:T14)  [unwired: 1 in, 1 out]
        n57 = Unbundle(w206) -> ("ROI"=w205:T18, "樣本比對參數R"=w186:T3, "Coordinate System Out"=w204:T13)
        n58 = Unbundle(w195) -> ("邊參數L"=w184:T1, "ROI"=w194:T18)
        n59 = Unbundle(w177) -> ("邊參數R"=w175:T1, "ROI"=w176:T18)
        n60 = call "Image FGV.vi"("Image action"=Image_action."讀取圖片", "圖片名稱"="Pattern_R") -> ("Image Out"=w211:T5)  [unwired: 8 in, 1 out]
        n61 = call "浪代_Match_Sub.vi"("樣本比對參數"=w186, "ROI Descriptor"=w205, "Mode"=w210, "error in (no error)"=w209, "Coordinate System In"=w204, "Template Image"=w211, "Image"=w201) -> ("error out"=w183:errorcluster, "Coordinate System Out"=w174:T13)  [unwired: 2 in, 1 out]
        n62 = call "浪代_Line_Sub.vi"("邊參數"=w184, "error in (no error)"=w183, "ROI"=w194, "Coordinate System"=w193, "Image"=w201) -> ("error out"=w179:errorcluster, "Image Out"=w178:T5)  [unwired: 4 in, 1 out]
        n63 = call "浪代_Line_Sub.vi"("邊參數"=w175, "error in (no error)"=w179, "ROI"=w176, "Coordinate System"=w174, "Image"=w178) -> ()  [unwired: 4 in, 3 out]
      }
      frame "             4.2.1浪代-Pattern_L" {
        w226 = 1 items=["All", "Low Discrepancy Sampling", "Grayscale Value Pyramid", "Gradients Pyramid"] ("Algorithm")
        n64 = call "Image FGV.vi"("Image action"=Image_action."讀取圖片", "圖片名稱"="Pattern_L") -> ("Image Out"=w227:T5)  [unwired: 8 in, 1 out]
        n65 = call "Image FGV.vi"("Image action"=Image_action."讀取圖片", "圖片名稱"="Image") -> ("Image Out"=w228:T5)  [unwired: 8 in, 1 out]
        n66 = property on="Image" class="ImageControl"() -> ("ROI"=w225:T18)  [unwired: 2 in, 2 out]
        n67 = call "浪代_Pattern_Sub.vi"("Algorithm"=w226, "ROI"=w225, "Image Dst"=w227, "Image Src"=w228) -> ()  [unwired: 6 in, 2 out]
        n68 = Enqueue Element(queue=w237, element=Setting_Control_Main_Action."       3.2影像-更新影像", error in (no error)=w235) -> (queue out=w236:refnum<queue>, error out=w234:errorcluster)  [unwired: 1 in, 1 out]
      }
      frame "             4.2.2浪代-Match_L" {
        w256 = u16 0 items=["Find Reference", "Update CoordSys"] ("Mode")
        n69 = property on="Image" class="ImageControl"() -> ("ROI"=w246:T18)  [unwired: 2 in, 2 out]
        n70 = call "Image FGV.vi"("Image action"=Image_action."讀取圖片", "圖片名稱"="Pattern_L") -> ("Image Out"=w255:T5)  [unwired: 8 in, 1 out]
        n71 = call "Image FGV.vi"("Image action"=Image_action."讀取圖片", "圖片名稱"="Image") -> ("Image Out"=w257:T5)  [unwired: 8 in, 1 out]
        n72 = call "浪代_Match_Sub.vi"("樣本比對參數"="樣本比對參數L", "ROI Descriptor"=w246, "Mode"=w256, "Coordinate System In"=T13 {"Reference System"={"Origin"={"X"=0.0, "Y"=0.0}, "Angle (deg)"=0.0, "Axis Reference"=0}, "Measurement System"={"Origin"={"X"=0.0, "Y"=0.0}, "Angle (deg)"=0.0, "Axis Reference"=0}}, "Template Image"=w255, "Image"=w257) -> ("Coordinate System Out"=w247:T13)  [unwired: 3 in, 2 out]
        n73 = local read "檢測項目"() -> (w241:T4)
        n74 = property on="檢測項目" class="Enum (strict)"() -> ("Strings []"=w243:string[])  [unwired: 2 in, 2 out]
        n75 = To Long Integer(number=w241) -> (32bit integer=w242:i32)
        n76 = Bundle("樣本比對參數L"="樣本比對參數L", "ROI"=w246, "Coordinate System Out"=w247) -> (w245:T15)  [unwired: 1 in]
        n77 = Index Array(array=w243, index=w242) -> (element=w239:string)
        n78 = To Variant(anything=w245) -> (Variant=w244:variant)
        n79 = Enqueue Element(queue=w253, element=Setting_Control_Main_Action."       3.2影像-更新影像", error in (no error)=w251) -> (queue out=w252:refnum<queue>, error out=w250:errorcluster)  [unwired: 1 in, 1 out]
        n80 = Bundle(w239, "Variant"=w244) -> (w240:cluster{string, "Variant":variant})  [unwired: 1 in]
        n81 = call "Main_FGV_Data.vi"("Action_Data"=Action_Data."Set Data", "Data In"=w240, "Data name"=w239) -> ()  [unwired: 7 in, 2 out]
      }
      frame "             4.2.3浪代-Pattern_R" {
        w268 = 1 items=["All", "Low Discrepancy Sampling", "Grayscale Value Pyramid", "Gradients Pyramid"] ("Algorithm")
        n82 = call "Image FGV.vi"("Image action"=Image_action."讀取圖片", "圖片名稱"="Pattern_R") -> ("Image Out"=w269:T5)  [unwired: 8 in, 1 out]
        n83 = call "Image FGV.vi"("Image action"=Image_action."讀取圖片", "圖片名稱"="Image") -> ("Image Out"=w270:T5)  [unwired: 8 in, 1 out]
        n84 = property on="Image" class="ImageControl"() -> ("ROI"=w267:T18)  [unwired: 2 in, 2 out]
        n85 = call "浪代_Pattern_Sub.vi"("Algorithm"=w268, "ROI"=w267, "Image Dst"=w269, "Image Src"=w270) -> ()  [unwired: 6 in, 2 out]
        n86 = Enqueue Element(queue=w265, element=Setting_Control_Main_Action."       3.2影像-更新影像", error in (no error)=w264) -> (queue out=w266:refnum<queue>, error out=w263:errorcluster)  [unwired: 1 in, 1 out]
      }
      frame "             4.2.4浪代-Match_R" {
        w293 = u16 0 items=["Find Reference", "Update CoordSys"] ("Mode")
        n87 = property on="Image" class="ImageControl"() -> ("ROI"=w283:T18)  [unwired: 2 in, 2 out]
        n88 = call "Image FGV.vi"("Image action"=Image_action."讀取圖片", "圖片名稱"="Pattern_R") -> ("Image Out"=w292:T5)  [unwired: 8 in, 1 out]
        n89 = call "Image FGV.vi"("Image action"=Image_action."讀取圖片", "圖片名稱"="Image") -> ("Image Out"=w294:T5)  [unwired: 8 in, 1 out]
        n90 = call "浪代_Match_Sub.vi"("樣本比對參數"="樣本比對參數R", "ROI Descriptor"=w283, "Mode"=w293, "Coordinate System In"=T13 {"Reference System"={"Origin"={"X"=0.0, "Y"=0.0}, "Angle (deg)"=0.0, "Axis Reference"=0}, "Measurement System"={"Origin"={"X"=0.0, "Y"=0.0}, "Angle (deg)"=0.0, "Axis Reference"=0}}, "Template Image"=w292, "Image"=w294) -> ("Coordinate System Out"=w284:T13)  [unwired: 3 in, 2 out]
        n91 = local read "檢測項目"() -> (w278:T4)
        n92 = property on="檢測項目" class="Enum (strict)"() -> ("Strings []"=w280:string[])  [unwired: 2 in, 2 out]
        n93 = Bundle("ROI"=w283, "樣本比對參數R"="樣本比對參數R", "Coordinate System Out"=w284) -> (w282:T14)  [unwired: 1 in]
        n94 = To Long Integer(number=w278) -> (32bit integer=w279:i32)
        n95 = Index Array(array=w280, index=w279) -> (element=w277:string)
        n96 = To Variant(anything=w282) -> (Variant=w281:variant)
        n97 = Enqueue Element(queue=w290, element=Setting_Control_Main_Action."       3.2影像-更新影像", error in (no error)=w289) -> (queue out=w288:refnum<queue>, error out=w287:errorcluster)  [unwired: 1 in, 1 out]
        n98 = Bundle(w277, "Variant"=w281) -> (w276:cluster{string, "Variant":variant})  [unwired: 1 in]
        n99 = call "Main_FGV_Data.vi"("Action_Data"=Action_Data."Set Data", "Data In"=w276, "Data name"=w277) -> ()  [unwired: 7 in, 2 out]
      }
      frame "             4.2.5檢測-找邊_L" {
        n100 = property on="Image" class="ImageControl"() -> ("ROI"=w304:T18)  [unwired: 2 in, 2 out]
        n101 = call "Image FGV.vi"("Image action"=Image_action."讀取圖片", "圖片名稱"="Image") -> ("Image Out"=w310:T5)  [unwired: 8 in, 1 out]
        n102 = call "浪代_Line_Sub.vi"("邊參數"="邊參數L", "ROI"=w304, "Coordinate System"=T13 {"Reference System"={"Origin"={"X"=0.0, "Y"=0.0}, "Angle (deg)"=0.0, "Axis Reference"=0}, "Measurement System"={"Origin"={"X"=0.0, "Y"=0.0}, "Angle (deg)"=0.0, "Axis Reference"=0}}, "Image"=w310) -> ()  [unwired: 5 in, 3 out]
        n103 = local read "檢測項目"() -> (w306:T4)
        n104 = property on="檢測項目" class="Enum (strict)"() -> ("Strings []"=w307:string[])  [unwired: 2 in, 2 out]
        n105 = Bundle("邊參數L"="邊參數L", "ROI"=w304) -> (w303:T12)  [unwired: 1 in]
        n106 = To Long Integer(number=w306) -> (32bit integer=w305:i32)
        n107 = To Variant(anything=w303) -> (Variant=w302:variant)
        n108 = Index Array(array=w307, index=w305) -> (element=w300:string)
        n109 = Bundle(w300, "Variant"=w302) -> (w301:cluster{string, "Variant":variant})  [unwired: 1 in]
        n110 = Enqueue Element(queue=w317, element=Setting_Control_Main_Action."       3.2影像-更新影像", error in (no error)=w316) -> (queue out=w315:refnum<queue>, error out=w314:errorcluster)  [unwired: 1 in, 1 out]
        n111 = call "Main_FGV_Data.vi"("Action_Data"=Action_Data."Set Data", "Data In"=w301, "Data name"=w300) -> ()  [unwired: 7 in, 2 out]
      }
      frame "             4.2.6檢測-找邊_R" {
        n112 = property on="Image" class="ImageControl"() -> ("ROI"=w328:T18)  [unwired: 2 in, 2 out]
        n113 = call "Image FGV.vi"("Image action"=Image_action."讀取圖片", "圖片名稱"="Image") -> ("Image Out"=w334:T5)  [unwired: 8 in, 1 out]
        n114 = call "浪代_Line_Sub.vi"("邊參數"="邊參數R", "ROI"=w328, "Coordinate System"=T13 {"Reference System"={"Origin"={"X"=0.0, "Y"=0.0}, "Angle (deg)"=0.0, "Axis Reference"=0}, "Measurement System"={"Origin"={"X"=0.0, "Y"=0.0}, "Angle (deg)"=0.0, "Axis Reference"=0}}, "Image"=w334) -> ()  [unwired: 5 in, 3 out]
        n115 = local read "檢測項目"() -> (w330:T4)
        n116 = property on="檢測項目" class="Enum (strict)"() -> ("Strings []"=w331:string[])  [unwired: 2 in, 2 out]
        n117 = Bundle("邊參數R"="邊參數R", "ROI"=w328) -> (w327:T11)  [unwired: 1 in]
        n118 = To Long Integer(number=w330) -> (32bit integer=w329:i32)
        n119 = To Variant(anything=w327) -> (Variant=w326:variant)
        n120 = Index Array(array=w331, index=w329) -> (element=w324:string)
        n121 = Bundle(w324, "Variant"=w326) -> (w325:cluster{string, "Variant":variant})  [unwired: 1 in]
        n122 = Enqueue Element(queue=w323, element=Setting_Control_Main_Action."       3.2影像-更新影像", error in (no error)=w320) -> (queue out=w322:refnum<queue>, error out=w319:errorcluster)  [unwired: 1 in, 1 out]
        n123 = call "Main_FGV_Data.vi"("Action_Data"=Action_Data."Set Data", "Data In"=w325, "Data name"=w324) -> ()  [unwired: 7 in, 2 out]
      }
      frame "5.0功能-雷射控制" {
      }
      frame "      5.1雷射-初始化" {
      }
      frame "      5.2雷射-寫入數值" {
      }
      frame "      5.3雷射-讀出數值" {
      }
      frame "      5.4雷射-雷射觸發" {
      }
      frame "      5.5雷射-關閉" {
      }
      frame "6.0功能-檔案" {
      }
      frame "       6.1檔案-初始化" {
        n124 = call "Main_FGV_Data.vi"("Action_Data"=Action_Data."Initialize") -> ()  [unwired: 9 in, 2 out]
      }
      frame "       6.2檔案-儲存檔案" {
        w360 = "Pattern_R" ("圖片名稱")
        w363 = "Pattern_L" ("圖片名稱")
        w365 = path "C:/Users/noname/Desktop/Main-Page/四穴雷切/Data資料夾/setting Data" ("file (use dialog)")
        n125 = property on="物料名稱" class="Enum (strict)"() -> ("Strings []"=w357:string[])  [unwired: 2 in, 2 out]
        n126 = To Long Integer(number="物料名稱") -> (32bit integer=w355:i32)
        n127 = Index Array(array=w357, index=w355) -> (element=w354:string)
        n128 = call "Image FGV.vi"("Image action"=Image_action."讀取圖片", "圖片名稱"=w360) -> ("error out"=w373:errorcluster, "Image Out"=w372:T5)  [unwired: 8 in]
        n129 = call "Image FGV.vi"("Image action"=Image_action."讀取圖片", "圖片名稱"=w363) -> ("error out"=w374:errorcluster, "Image Out"=w375:T5)  [unwired: 8 in]
        n130 = Concatenate Strings(w354, "Data" ("string")) -> (w358:string)
        n131 = call "Main_FGV_Data.vi"("Action_Data"=Action_Data."Idle") -> ("Data Array out"=w378:cluster{"Data name":string, "Data":variant}[])  [unwired: 9 in, 1 out]
        n132 = Concatenate Strings(w358, "-" ("string"), w360, ".png" ("string")) -> (w367:string)
        n133 = Build Path(base path=w365, name or relative path=w358) -> (appended path=w371:path)
        n134 = Concatenate Strings(w358, "-" ("string"), w363, ".png" ("string")) -> (w370:string)
        n135 = Build Path(base path=w365, name or relative path=w367) -> (appended path=w362:path)
        n136 = Build Path(base path=w365, name or relative path=w370) -> (appended path=w366:path)
        n137 = Write to Binary File(file (use dialog)=w371, data=w378) -> ()  [unwired: 4 in, 3 out]
        n138 = call "IMAQ Write Image And Vision Info File 2"("error in (no error)"=w373, "File Path"=w362, "Image"=w372) -> ()  [unwired: 7 in, 2 out]
        n139 = call "IMAQ Write Image And Vision Info File 2"("error in (no error)"=w374, "File Path"=w366, "Image"=w375) -> ()  [unwired: 7 in, 2 out]
      }
      frame "       6.3檔案-開啟檔案" {
        n140 = call "Image FGV.vi"("Image action"=Image_action."讀取圖片", "圖片名稱"="Pattern_L") -> ("Image Out"=w405:T5)  [unwired: 8 in, 1 out]
        n141 = call "Image FGV.vi"("Image action"=Image_action."讀取圖片", "圖片名稱"="Pattern_R") -> ("Image Out"=w398:T5)  [unwired: 8 in, 1 out]
        n142 = call "Main_FGV_Data.vi"("Action_Data"=Action_Data."Initialize") -> ("Data Array out"=w412:cluster{"Data name":string, "Data":variant}[])  [unwired: 9 in, 1 out]
        n143 = call "File Dialog"("start path"=path "C:/Users/noname/Desktop/Main-Page/四穴雷切/Data資料夾/setting Data") -> ("selected path"=w387:path, "error out"=w383:errorcluster)  [unwired: 11 in, 2 out]
        n144 = Strip Path(path=w387) -> (stripped path=w388:path, name=w389:string)
        n145 = Strip Path(path=w387) -> (stripped path=w386:path, name=w385:string)
        n146 = Read from Binary File(5:w412, 11:w387) -> (0:w382:errorcluster, 2:w407:cluster{"Data name":string, "Data":variant}[])  [unwired: 4 in, 2 out]
        n147 = Concatenate Strings(w389, "-" ("string"), "Pattern_L.png" ("name or relative path")) -> (w392:string)
        n148 = Concatenate Strings(w385, "-" ("string"), "Pattern_R.png" ("name or relative path")) -> (w391:string)
        n149 = Build Path(base path=w388, name or relative path=w392) -> (appended path=w406:path)
        n150 = Build Path(base path=w386, name or relative path=w391) -> (appended path=w399:path)
        n151 = for {
          tunnel: w407 -> [w414] mode=indexing
          n152 = Unbundle(w414) -> ("Data name"=w415:string)  [unwired: 1 out]
          n153 = call "Main_FGV_Data.vi"("Action_Data"=Action_Data."Set Data", "Data In"=w414, "Data name"=w415) -> ()  [unwired: 7 in, 2 out]
        }
        n154 = call "IMAQ Read Image And Vision Info"("File Path"=w406, "Image"=w405) -> ("error out"=w397:errorcluster)  [unwired: 7 in, 2 out]
        n155 = call "IMAQ Read Image And Vision Info"("File Path"=w399, "Image"=w398) -> ("error out"=w396:errorcluster)  [unwired: 7 in, 2 out]
        n156 = Enqueue Element(queue=w404, element=Setting_Control_Main_Action."       3.2影像-更新影像", error in (no error)=w403) -> (queue out=w402:refnum<queue>, error out=w401:errorcluster)  [unwired: 1 in, 1 out]
      }
      frame "7.0 錯誤" {
      }
      frame "8.0等待" {
      }
      frame "       8.1等待(計算時間)" {
      }
      frame "9.0離開" {
      }
      frame "10.0功能-機台驗證" {
      }
      frame "      10.1機台驗證-初始化" {
      }
      frame "      10.2機台驗證-檢測" {
      }
      frame "11.0對話視窗" {
      }
    }
  }
  n157 = while {
    tunnel: w8 -> [w439]
    tunnel: w7 -> [w438]
    stop <- w437 stop-if-true
    n158 = event shown="[7] \"離開\": Value Change" {
      selector: _ -> [_ _ _ _ _ _ _ _]
      dyn-events: _ -> [_ _ _ _ _ _ _ _]
      timeout: _ -> [_ _ _ _ _ _ _ _]
      tunnel: w439 -> [w441 w443 w447 w452 w474 w477 w480 w483]
      tunnel: [w441 w443 w447 w453 w474 w477 w480 w483] -> w436
      tunnel: w438 -> [w440 w442 w446 w450 w473 w476 w479 w482]
      tunnel: [w440 w442 w446 w451 w473 w476 w479 w482] -> w434
      tunnel: [_ _ _ _ _ _ _ TRUE] -> w437
      tunnel: [_ Setting_Control_Main_Action."二、動作-單次取像" ("element") Setting_Control_Main_Action."三、動作-連續取像" ("element") w449 Setting_Control_Main_Action."四、動作-單步測試" ("element") Setting_Control_Main_Action."五、動作-連續測試" ("element") Setting_Control_Main_Action."       8.1等待(計算時間)" ("element") Setting_Control_Main_Action."六、動作-離開" ("element")] -> w435
      event Timeout {
        n159 = event-data() -> ()  [unwired: 1 in, 3 out]
      }
      event "取像": Value Change {
        n160 = event-data() -> ()  [unwired: 1 in, 1 out]
      }
      event "連續取像": Value Change {
        n161 = event-data() -> ()  [unwired: 1 in, 1 out]
      }
      event "確認檢測項目": Value Change {
        n162 = event-data() -> ()  [unwired: 1 in, 1 out]
        n163 = local read "檢測項目"() -> (w448:T4)
        n164 = case shown="\"Pattern_R\"" w448 {
          tunnel: [w456 w459 w462 w465 w468 w471] -> w453
          tunnel: w452 -> [w456 w459 w462 w465 w468 w471]
          tunnel: [w455 w458 w461 w464 w467 w470] -> w451
          tunnel: w450 -> [w455 w458 w461 w464 w467 w470]
          tunnel: [Setting_Control_Main_Action."             4.2.1浪代-Pattern_L" ("element") Setting_Control_Main_Action."             4.2.2浪代-Match_L" ("element") Setting_Control_Main_Action."             4.2.3浪代-Pattern_R" ("element") Setting_Control_Main_Action."             4.2.4浪代-Match_R" ("element") Setting_Control_Main_Action."             4.2.5檢測-找邊_L" ("element") Setting_Control_Main_Action."             4.2.6檢測-找邊_R" ("element")] -> w449
          frame "Pattern_L", Default {
          }
          frame "Match_L" {
          }
          frame "Pattern_R" {
          }
          frame "Match_R" {
          }
          frame "找邊_L" {
          }
          frame "找邊R" {
          }
        }
      }
      event "單步測試": Value Change {
        n165 = event-data() -> ()  [unwired: 1 in, 1 out]
      }
      event "連續測試": Value Change {
        n166 = event-data() -> ()  [unwired: 1 in, 1 out]
      }
      event Value Change {
        n167 = event-data() -> ()  [unwired: 1 in, 2 out]
      }
      event "離開": Value Change {
        n168 = event-data() -> ()  [unwired: 1 in, 1 out]
      }
    }
    n169 = Enqueue Element(queue=w436, element=w435, error in (no error)=w434) -> ()  [unwired: 1 in, 3 out]
  }
  n170 = Multiply(x=cluster{"Width":u32, "Height":u32} {"Width"=715, "Height"=565} ("Image Area:Size:All Elements"), y=1.0) -> (x*y=w2:cluster{"Width":dbl, "Height":dbl})
  n171 = property on="Image" class="ImageControl"("Image Area Size"=w2) -> ()  [unwired: 2 in, 2 out]
  n172 = Release Queue(queue=w6, error in (no error)=w5) -> ()  [unwired: 1 in, 3 out]
